vi "setUp.vi"(8 "error in (no error)":errorcluster, 11 "VI in":refnum<vi>) -> (0 "error out":errorcluster, 3 "fpMgr out":refnum<class "fpMgr.lvclass">)   [LabVIEW 2019, in "LabVIEW-ProviderShell.lvlib" / "fpMgr.lvclass"]
uses:
  fpMgr.lvclass
  def-ConnectorInfo.ctl
  fpMgr.lvclass/fpMgr.ctl
  7d342f29-83a4-4e21-81e0-3669ec85bedb.vi
  14c89cb6-dc9d-4114-91f1-592d8beb9791.vi
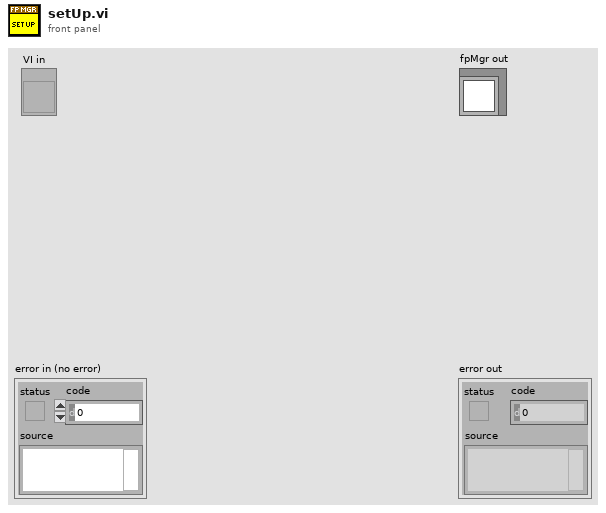
[diagram p1: front panel]
types:
  T1 = typedef "LabVIEW-ProviderShell.lvlib/fpMgr.lvclass/def-ConnectorInfo.ctl" = cluster{"Value":variant, "Label.Text":string, "error":errorcluster, "DatatypeDescription":string, "Indicator":bool}
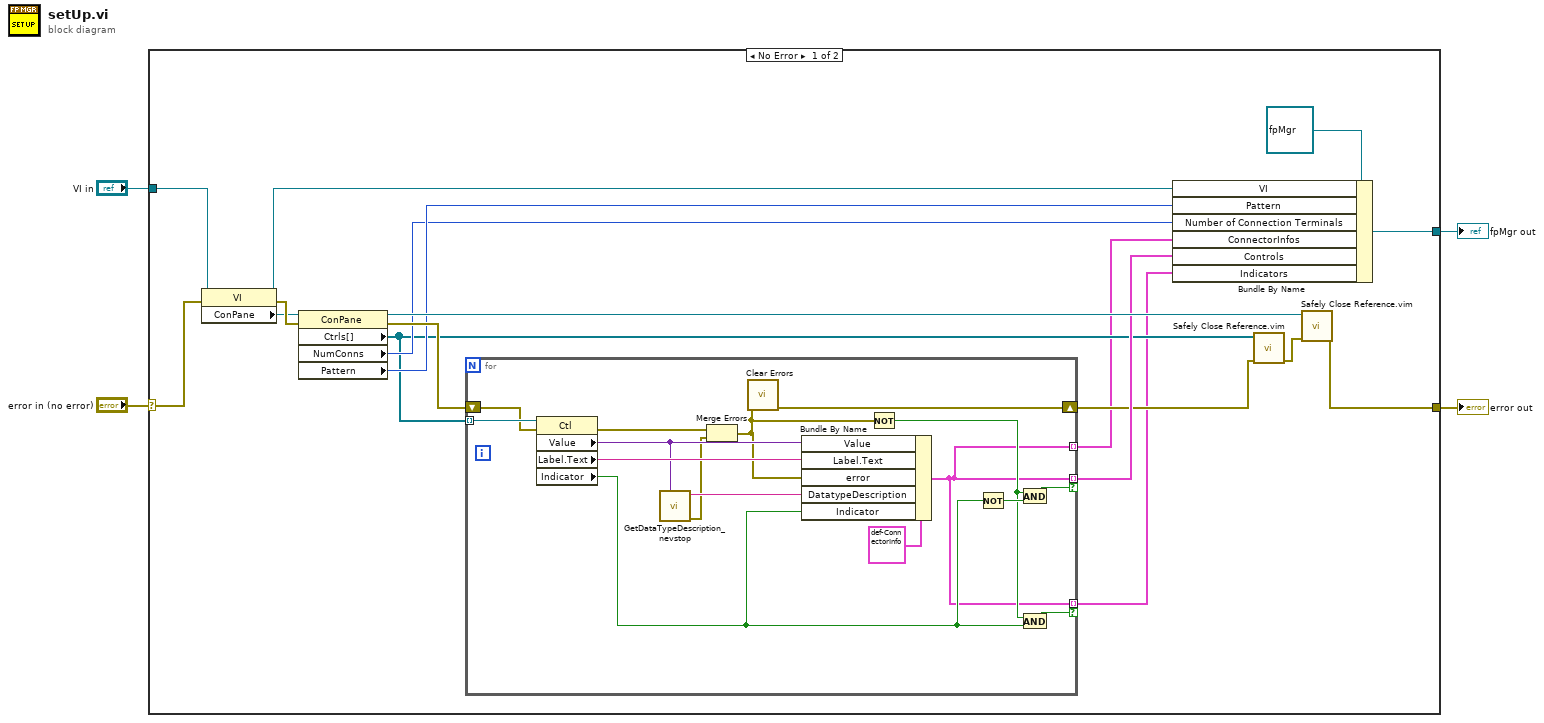
[diagram p0: block diagram]
diagram:
  n1 = case shown="No Error" "error in (no error)" {
    selector: "error in (no error)" -> [w19 w39]
    tunnel: [w21 w39] -> w3
    tunnel: "VI in" -> [w16 _]
    tunnel: [w10 _] -> w1
    frame No Error {
      n2 = property on="Property Node" class="VI"(reference=w16, error in=w19) -> (reference out=w14:refnum<vi>, error out=w18:errorcluster, "ConPane"=w17:refnum<vi>)
      n3 = property on="Property Node" class="ConPane"(reference=w17, error in=w18) -> (reference out=w22:refnum<vi>, error out=w20:errorcluster, "Ctrls[]"=w9:refnum<vi>[], "NumConns"=w11:u32, "Pattern"=w12:u32)
      n4 = for {
        tunnel: w9 -> [w38] mode=indexing
        shift-right: [w36] -> w7
        shift-left: w20 -> [w37]
        tunnel: [w23] -> w13 mode=indexing if=w26
        tunnel: [w23] -> w6 mode=indexing if=w27
        tunnel: [w23] -> w5 mode=indexing
        n5 = property class="Ctl"(reference=w38, error in=w37) -> (error out=w33:errorcluster, "Value"=w32:variant, "Label.Text"=w34:string, "Indicator"=w29:bool)  [unwired: 1 out]
        n6 = call <userlib>:"GetDataTypeDescription_nevstop.vi"("Variant"=w32) -> ("error out"=w30:errorcluster, "String"=w31:string)  [unwired: 9 in]
        n7 = Merge Errors(w33, w30) -> (w25:errorcluster)
        n8 = call <vilib>:"Clear Errors.vi"("error in (no error)"=w25) -> ("error out"=w36:errorcluster)  [unwired: 5 in, 1 out]
        n9 = Bundle By Name(cluster=T1 {"Value"=variant, "Label.Text"="", "error"={"status"=FALSE, "code"=0, "source"=""}, "DatatypeDescription"="", "Indicator"=FALSE} ("Cluster"), "Value"=w32, "Label.Text"=w34, "error"=w25, "DatatypeDescription"=w31, "Indicator"=w29) -> (w23:T1)
        n10 = Not(x=w25) -> (.not. x?=w24:bool)
        n11 = Not(x=w29) -> (.not. x?=w28:bool)
        n12 = And(x=w24, y=w28) -> (x .and. y?=w26:bool)
        n13 = And(x=w24, y=w29) -> (x .and. y?=w27:bool)
      }
      n14 = Bundle By Name(cluster=refnum<class "fpMgr.lvclass"> refnum ("LabVIEW-ProviderShell.lvlib:fpMgr.lvclass"), "VI"=w14, "Pattern"=w12, "Number of Connection Terminals"=w11, "ConnectorInfos"=w5, "Controls"=w13, "Indicators"=w6) -> (w10:refnum<class "fpMgr.lvclass">)
      n15 = call "Safely Close Reference.vim"("error in (no error)"=w7, "LVClassLibrary in"=w9) -> ("error out"=w8:errorcluster)  [unwired: 9 in]
      n16 = call "Safely Close Reference.vim"("error in (no error)"=w8, "LVClassLibrary in"=w22) -> ("error out"=w21:errorcluster)  [unwired: 9 in]
    }
    frame Error {
    }
  }
  "error out" <- w3
  "fpMgr out" <- w1
